vi "Control Panel.vi"(8 "error in (no error)":errorcluster, 11 "Keithley Multimeter in":refnum<class "Testing Keithley Multimeter.lvclass">) -> (0 "error out":errorcluster, 3 "Keithley Multimeter out":refnum<class "Testing Keithley Multimeter.lvclass">)   [LabVIEW 2017, in "Testing Keithley Multimeter.lvclass"]
doc: "(Dynamic) A user-level application that simulates the physical front panel of the Instrument. Provide the user with buttons to manually control features of the instrument, and provide indicators of its current state."
uses:
  Testing Keithley Multimeter.lvclass
panel:
  in  "Keithley Values":T1={"range (auto:0)"=0, "range value (volts)"=1000.0, "resolution (4.5 digits:3)"=3, "integration time (0:auto)"=0, "integ. value"=0.01667, "digital filter (off:0)"=0, "advanced filter (off:0)"=0, "dig. filter count"=10.0, "reference (off:0)"=0, "reference value (volts)"=0.0, "noise tolerance (%)"=1.0} {"noise tolerance (%)" min=0.0 max=100.0 step=1.0 format="%^.2e"; "reference value (volts)" min=-1100.0 max=1100.0 format="%^.2e"; "reference (off:0)" items=["off", "set reference value"]; "dig. filter count" min=1.0 max=100.0 step=1.0 format="%^.2e"; "advanced filter (off:0)" items=["off", "enabled"]; "digital filter (off:0)" items=["off", "auto filter", "auto filter once", "moving filter", "repeating filter"]; "integ. value" format="%^.2e"; "integration time (0:auto)" items=["automatic", "automatic once", "set to minimum", "set to maximum", "set aperature value", "set NPLC value"]; "resolution (4.5 digits:3)" items=["auto resolution", "auto resolution once", "3.5 digits", "4.5 digits", "5.5 digits", "6.5 digits", "7.5 digits", "8.5 digits"]; "range (auto:0)" items=["autorange", "autorange once", "set min range", "set max range", "set range value"]; "range value (volts)" min=0.2 max=1000.0 format="%^.2e"}
  out "Unit":string="V"
  out "Current function":u16(ring)=1 items=["ac voltage", "dc voltage", "2-wire resistance", "4-wire resistance", "ac current", "dc current", "frequency", "temperature"]
  out "Tab Control":enum32{"0", "1", "2", "3", "4", "5", "6", "7"}(tab)
  in  "AC Voltage Configuration":T2={"dBm ref impedance (75:1)"=1, "peak window (secs)"=0.1, "detector (rms:0)"=0, "dB reference (volts)"=1.0, "AC voltage (volts:0)"=0, "reference value (volts)"=0.0, "range value (volts)"=750.0} {"range value (volts)" min=0.2 max=750.0 format="%^.2e"; "reference value (volts)" min=-775.0 max=775.0 format="%^.2e"; "AC voltage (volts:0)" items=["volts", "DB", "DBM"]; "dB reference (volts)" min=0.001 max=750.0 format="%.3f"; "detector (rms:0)" items=["RMS", "average", "low frequency RMS", "AC peak voltage", "DC negative peak spike", "DC positive peak spike"]; "peak window (secs)" min=0.1 max=9.9 format="%.2f"; "dBm ref impedance (75:1)" items=["50 ohms", "75 ohms", "93 ohms", "132 ohms", "300 ohms", "600 ohms"]}
  in  "DC Voltage Configuration":T3={"reference value (volts)"=0.0, "range value (volts)"=1000.0} {"range value (volts)" min=0.2 max=1000.0 format="%^.2e"; "reference value (volts)" min=-1100.0 max=1100.0 format="%^.2e"}
  in  "2 Wire Resistance Configuration":T4={"offset compensation"=FALSE, "reference value (ohms)"=0.0, "range value (ohms)"=1000000000.0} {"range value (ohms)" min=20.0 max=1000000000.0 format="%^.2e"; "reference value (ohms)" min=-1000000000.0 max=1000000000.0 format="%^.2e"}
  in  "4 Wire Resistance Configuration":T4={"offset compensation"=FALSE, "reference value (ohms)"=0.0, "range value (ohms)"=200000.0} {"range value (ohms)" min=20.0 max=200000.0 format="%^.2e"; "reference value (ohms)" min=-200000.0 max=200000.0 format="%^.2e"}
  in  "AC Current Configuration":T5={"detector (rms:0)"=0, "reference value (amps)"=0.0, "range value (amps)"=2.0} {"range value (amps)" min=0.0002 max=2.0 format="%^.2e"; "reference value (amps)" min=-2.1 max=2.1 format="%^.2e"; "detector (rms:0)" items=["RMS", "average"]}
  in  "DC Current Configuration":T6={"reference value (amps)"=0.0, "method"=TRUE, "range value (amps)"=2.0} {"range value (amps)" min=0.0002 max=2.0 format="%^.2e"; "reference value (amps)" min=-2.1 max=2.1 format="%^.2e"}
  in  "Frequency Configuration":T7={"source"=FALSE, "resolution (5 digits:1)"=1, "threshold current range (1mA:0)"=0, "reference value (Hz)"=0.0, "threshold current level"=0.0, "threshold voltage range (10V:1)"=1, "threshold voltage level"=0.0} {"threshold voltage level" min=-600.0 max=600.0 step=1.0 format="%^.2e"; "threshold voltage range (10V:1)" items=["1 V", "10 V", "100 V", "1000 V", "TTL"]; "threshold current level" min=-0.6 max=0.6 format="%^.2e"; "reference value (Hz)" min=0.0 max=15000000.0 format="%^.2e"; "threshold current range (1mA:0)" items=["1 mA", "10 mA", "100 mA", "1 A"]; "resolution (5 digits:1)" items=["4 digits", "5 digits"]}
  out "String":string
  in  "Configuration Values":T8={"range (auto:0)"=0, "dig. filter count"=10.0, "digital filter (off:0)"=0, "advanced filter (off:0)"=0, "integration time (0:auto)"=0, "integ. value"=0.01667, "resolution (4.5 digits:3)"=3, "noise tolerance (%)"=1.0, "reference (off:0)"=0, "coupling"=TRUE, "function (Vdc:1)"=1} {"function (Vdc:1)" items=["ac voltage", "dc voltage", "2-wire resistance", "4-wire resistance", "ac current", "dc current", "frequency", "temperature"]; "reference (off:0)" items=["off", "set reference value"]; "noise tolerance (%)" min=0.0 max=100.0 step=1.0 format="%^.2e"; "resolution (4.5 digits:3)" items=["auto resolution", "auto resolution once", "3.5 digits", "4.5 digits", "5.5 digits", "6.5 digits", "7.5 digits", "8.5 digits"]; "integ. value" format="%^.2e"; "integration time (0:auto)" items=["automatic", "automatic once", "set to minimum", "set to maximum", "set aperature value", "set NPLC value"]; "advanced filter (off:0)" items=["off", "enabled"]; "digital filter (off:0)" items=["off", "auto filter", "auto filter once", "moving filter", "repeating filter"]; "dig. filter count" min=1.0 max=100.0 step=1.0 format="%^.2e"; "range (auto:0)" items=["autorange", "autorange once", "set min range", "set max range", "set range value"]}
  in  "function (Vdc:1)":u16(ring)=1 items=["ac voltage", "dc voltage", "2-wire resistance", "4-wire resistance", "ac current", "dc current", "frequency", "temperature"]
  in  "Set":bool
  in  "Read":bool
  out "Output":dbl[](array[numeric])
  in  "Stop":bool
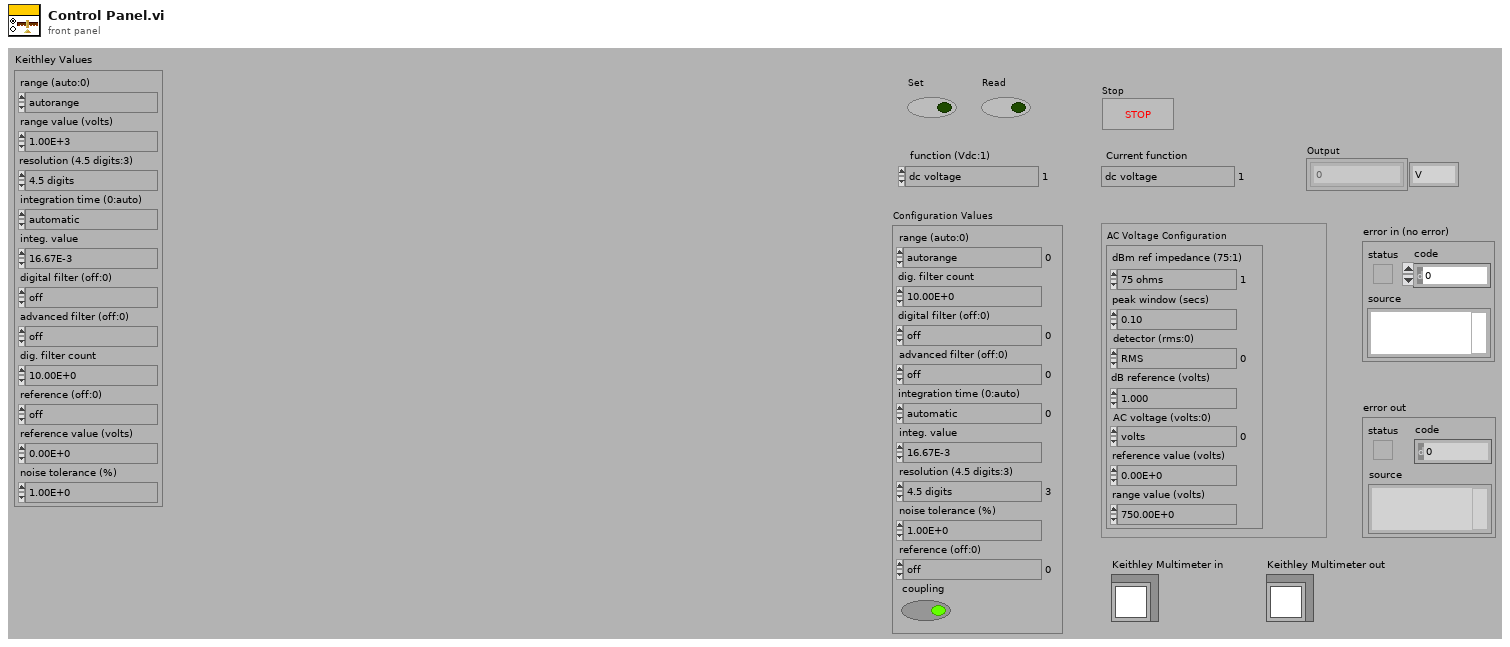
[diagram p1: front panel]
types:
  T1 = cluster{"range (auto:0)":u16, "range value (volts)":dbl, "resolution (4.5 digits:3)":u16, "integration time (0:auto)":u16, "integ. value":dbl, "digital filter (off:0)":u16, "advanced filter (off:0)":u16, "dig. filter count":dbl, "reference (off:0)":u16, "reference value (volts)":dbl, "noise tolerance (%)":dbl}
  T2 = cluster{"dBm ref impedance (75:1)":u16, "peak window (secs)":dbl, "detector (rms:0)":u16, "dB reference (volts)":dbl, "AC voltage (volts:0)":u16, "reference value (volts)":dbl, "range value (volts)":dbl}
  T3 = cluster{"reference value (volts)":dbl, "range value (volts)":dbl}
  T4 = cluster{"offset compensation":bool, "reference value (ohms)":dbl, "range value (ohms)":dbl}
  T5 = cluster{"detector (rms:0)":u16, "reference value (amps)":dbl, "range value (amps)":dbl}
  T6 = cluster{"reference value (amps)":dbl, "method":bool, "range value (amps)":dbl}
  T7 = cluster{"source":bool, "resolution (5 digits:1)":u16, "threshold current range (1mA:0)":u16, "reference value (Hz)":dbl, "threshold current level":dbl, "threshold voltage range (10V:1)":u16, "threshold voltage level":dbl}
  T8 = cluster{"range (auto:0)":u16, "dig. filter count":dbl, "digital filter (off:0)":u16, "advanced filter (off:0)":u16, "integration time (0:auto)":u16, "integ. value":dbl, "resolution (4.5 digits:3)":u16, "noise tolerance (%)":dbl, "reference (off:0)":u16, "coupling":bool, "function (Vdc:1)":u16}
  T9 = cluster{"error":bool, "code":i32, "source":string}
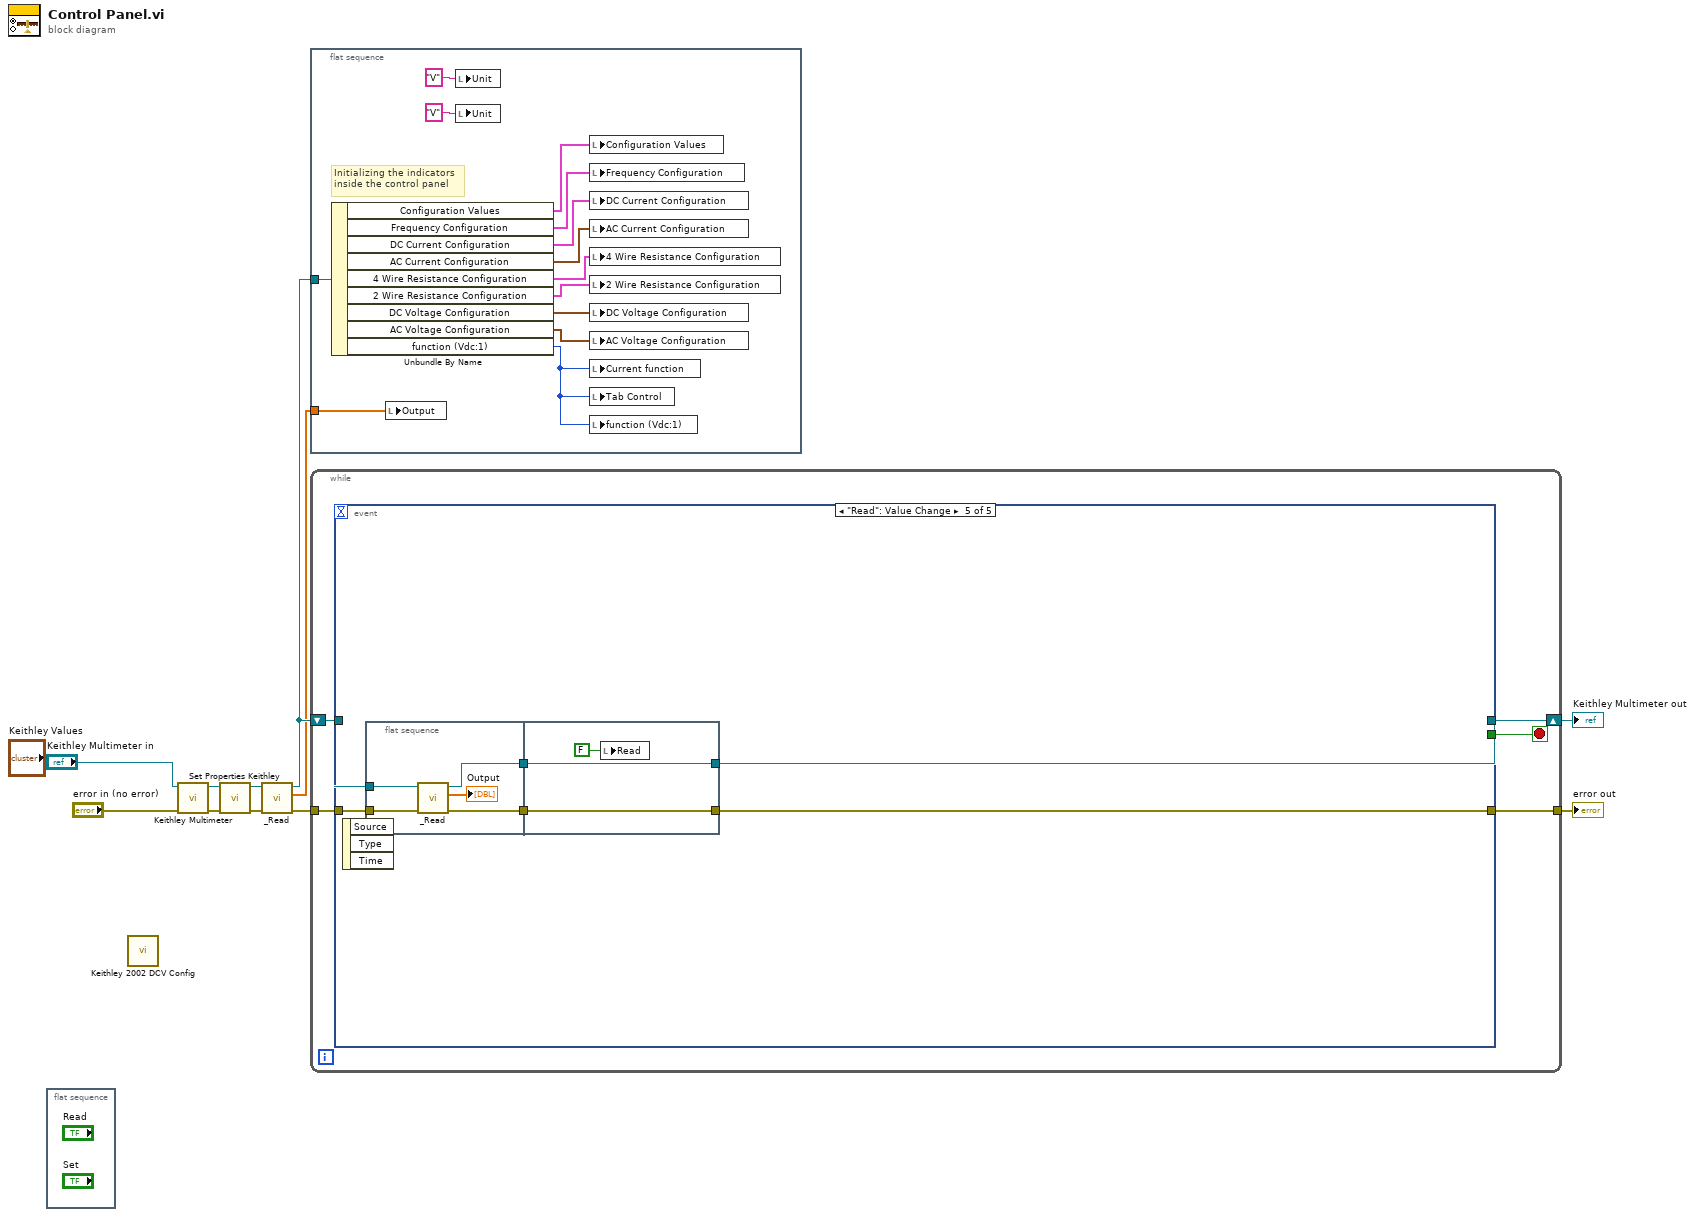
[diagram p0: block diagram]
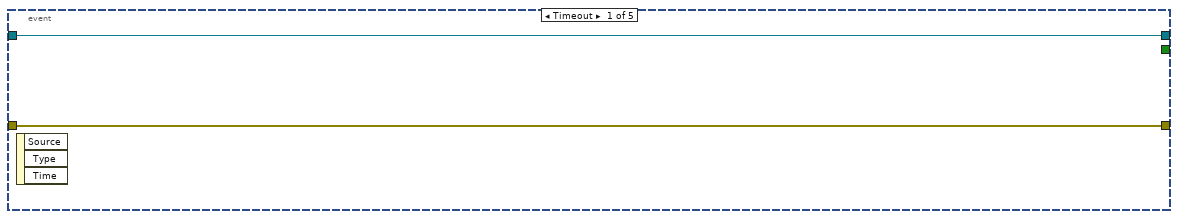
[diagram p2: hidden frame]
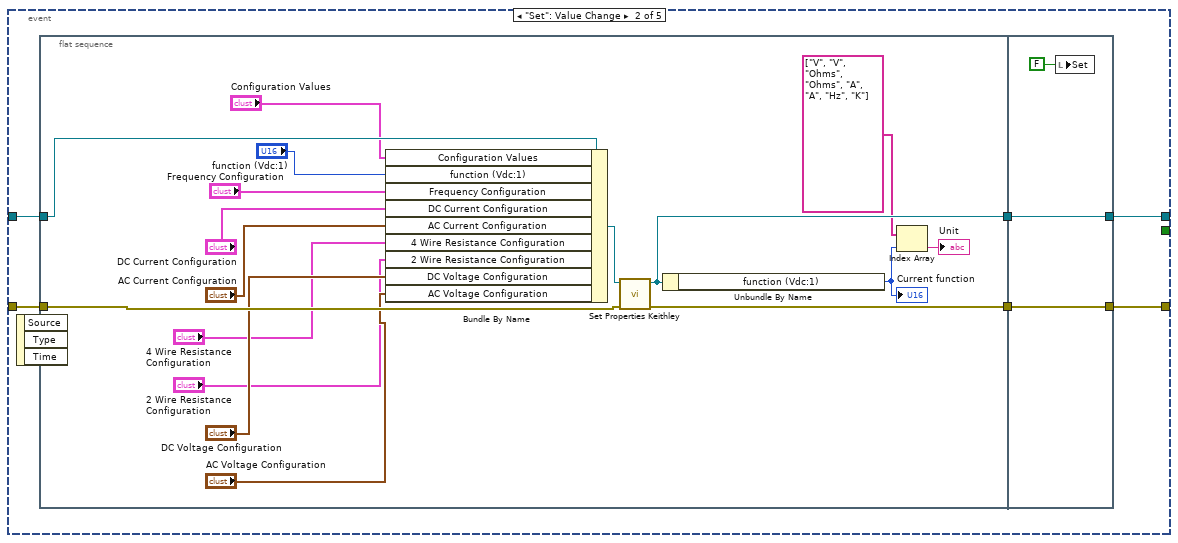
[diagram p3: hidden frame]
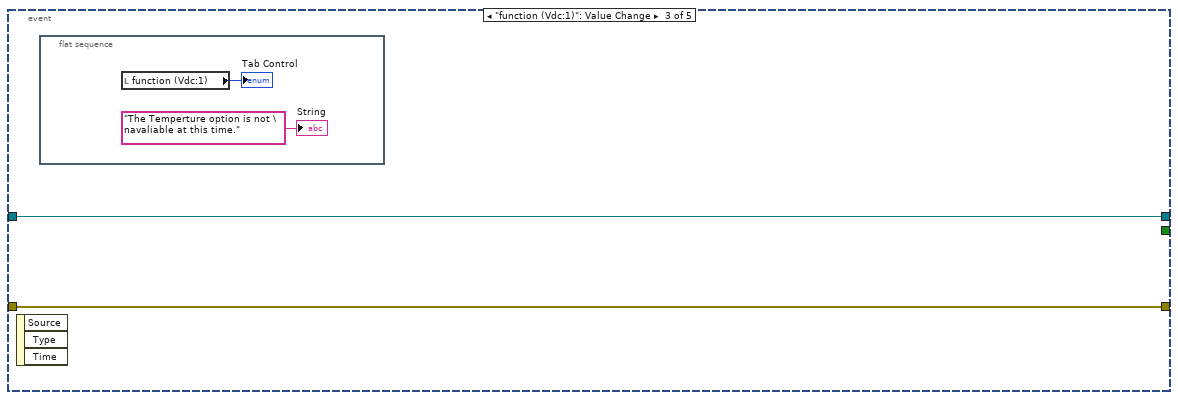
[diagram p4: hidden frame]
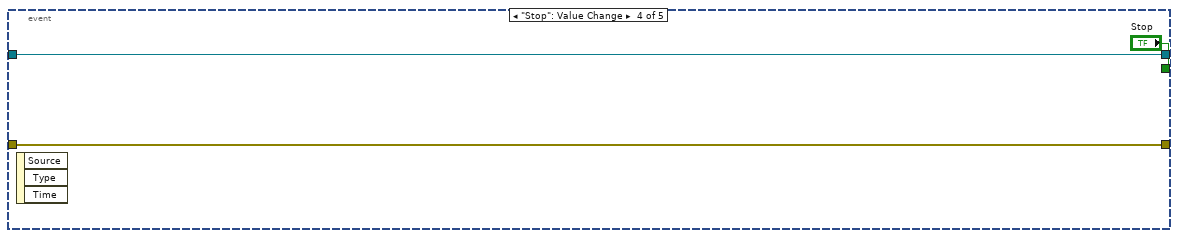
[diagram p5: hidden frame]
diagram:
  n1 = flat-sequence {
    frame #0 {
    }
  }
  n2 = call "Keithley 2002 DCV Config.vi"() -> ("GPIB address"=w11:string, "range value (volts)"=w10:dbl, "range (auto:0)"=w9:u16, "dig. filter count"=w8:dbl, "digital filter (off:0)"=w7:u16, "integ. value"=w6:dbl, "resolution (4.5 digits:3)"=w5:u16, "error in"=w4:T9, "reference (off:0)"=w3:u16, "reference value (volts)"=w2:dbl, "error out"=w1:T9)  [unwired: 5 in]
  n3 = call "Keithley Multimeter.vi"("error in (no error)"="error in (no error)", "Keithley Multimeter in"="Keithley Multimeter in") -> ("error out"=w18:errorcluster, "Keithley Multimeter out"=w17:refnum<class "Testing Keithley Multimeter.lvclass">)  [unwired: 8 in]
  n4 = call-dynamic "Set Properties Keithley.vi"("error in (no error)"=w18, "Keithley Multimeter in"=w17) -> ("error out"=w15:errorcluster, "Keithley Multimeter out"=w16:refnum<class "Testing Keithley Multimeter.lvclass">)  [unwired: 8 in]
  n5 = call-dynamic "_Read.vi"("error in (no error)"=w15, "Keithley Multimeter in"=w16) -> ("error out"=w14:errorcluster, "appended array"=w12:dbl[], "Keithley Multimeter out"=w13:refnum<class "Testing Keithley Multimeter.lvclass">)  [unwired: 7 in]
  n6 = flat-sequence {
    tunnel: w13 -> [w35]
    tunnel: w12 -> [w23]
    frame #0 {
      # "Initializing the indicators\ninside the control panel"
      n7 = Unbundle By Name(w35) -> ("Configuration Values"=w34:T8, "Frequency Configuration"=w33:T7, "DC Current Configuration"=w31:T6, "AC Current Configuration"=w32:T5, "4 Wire Resistance Configuration"=w30:T4, "2 Wire Resistance Configuration"=w29:T4, "DC Voltage Configuration"=w28:T3, "AC Voltage Configuration"=w27:T2, "function (Vdc:1)"=w24:u16)
      n8 = local write "Output"(w23) -> ()
      n9 = local write "Unit"("V" ("Unit")) -> ()
      n10 = local write "Unit"("V" ("Unit")) -> ()
      n11 = local write "Configuration Values"(w34) -> ()
      n12 = local write "Frequency Configuration"(w33) -> ()
      n13 = local write "DC Current Configuration"(w31) -> ()
      n14 = local write "AC Current Configuration"(w32) -> ()
      n15 = local write "4 Wire Resistance Configuration"(w30) -> ()
      n16 = local write "2 Wire Resistance Configuration"(w29) -> ()
      n17 = local write "DC Voltage Configuration"(w28) -> ()
      n18 = local write "AC Voltage Configuration"(w27) -> ()
      n19 = local write "Current function"(w24) -> ()
      n20 = local write "Tab Control"(w24) -> ()
      n21 = local write "function (Vdc:1)"(w24) -> ()
    }
  }
  n22 = while {
    tunnel: w14 -> [w40]
    tunnel: [w39] -> w22
    shift-right: [w38] -> w21
    shift-left: w13 -> [w36]
    stop <- w37 stop-if-true
    n23 = event shown="[4] \"Read\": Value Change" {
      selector: _ -> [_ _ _ _ _]
      dyn-events: _ -> [_ _ _ _ _]
      timeout: _ -> [_ _ _ _ _]
      tunnel: w40 -> [w41 w45 w70 w73 w81]
      tunnel: w36 -> [w42 w48 w69 w74 w80]
      tunnel: [w41 w46 w70 w73 w79] -> w39
      tunnel: [w42 w47 w69 w74 w78] -> w38
      tunnel: [_ _ _ "Stop" _] -> w37
      event Timeout {
        n24 = event-data() -> ()  [unwired: 1 in, 3 out]
      }
      event "Set": Value Change {
        n25 = event-data() -> ()  [unwired: 1 in, 3 out]
        n26 = flat-sequence {
          tunnel: w48 -> [w65]
          tunnel: w45 -> [w61]
          tunnel: [w64] -> w44
          tunnel: [w62] -> w43
          tunnel: [w67] -> w46
          tunnel: [w68] -> w47
          tunnel: w44 -> [w68]
          tunnel: w43 -> [w67]
          frame #0 {
            n27 = Bundle By Name(cluster=w65, "Configuration Values"="Configuration Values", "function (Vdc:1)"="function (Vdc:1)", "Frequency Configuration"="Frequency Configuration", "DC Current Configuration"="DC Current Configuration", "AC Current Configuration"="AC Current Configuration", "4 Wire Resistance Configuration"="4 Wire Resistance Configuration", "2 Wire Resistance Configuration"="2 Wire Resistance Configuration", "DC Voltage Configuration"="DC Voltage Configuration", "AC Voltage Configuration"="AC Voltage Configuration") -> (w63:refnum<class "Testing Keithley Multimeter.lvclass">)
            n28 = call-dynamic "Set Properties Keithley.vi"("error in (no error)"=w61, "Keithley Multimeter in"=w63) -> ("error out"=w62:errorcluster, "Keithley Multimeter out"=w64:refnum<class "Testing Keithley Multimeter.lvclass">)  [unwired: 8 in]
            n29 = Unbundle By Name(w64) -> ("function (Vdc:1)"=w49:u16)
            "Current function" <- w49
            n30 = Index Array(array=string[] ["V", "V", "Ohms", "Ohms", "A", "A", "Hz", "K"], index=w49) -> (element=→"Unit":string)
          }
          frame #1 {
            n31 = local write "Set"(FALSE ("Set")) -> ()
          }
        }
      }
      event "function (Vdc:1)": Value Change {
        n32 = event-data() -> ()  [unwired: 1 in, 3 out]
        n33 = flat-sequence {
          frame #0 {
            n34 = local read "function (Vdc:1)"() -> (→"Tab Control":u16)
            "String" <- "The Temperture option is not \navaliable at this time." ("String")
          }
        }
      }
      event "Stop": Value Change {
        n35 = event-data() -> ()  [unwired: 1 in, 3 out]
      }
      event "Read": Value Change {
        n36 = event-data() -> ()  [unwired: 1 in, 3 out]
        n37 = flat-sequence {
          tunnel: w81 -> [w86]
          tunnel: w80 -> [w85]
          tunnel: [w84] -> w77
          tunnel: [w82] -> w76
          tunnel: [w88] -> w78
          tunnel: [w89] -> w79
          tunnel: w77 -> [w89]
          tunnel: w76 -> [w88]
          frame #0 {
            n38 = call-dynamic "_Read.vi"("error in (no error)"=w86, "Keithley Multimeter in"=w85) -> ("error out"=w84:errorcluster, "appended array"=→"Output":dbl[], "Keithley Multimeter out"=w82:refnum<class "Testing Keithley Multimeter.lvclass">)  [unwired: 7 in]
          }
          frame #1 {
            n39 = local write "Read"(FALSE ("Read")) -> ()
          }
        }
      }
    }
  }
  "error out" <- w22
  "Keithley Multimeter out" <- w21
